vi "rszvl Initiate.vi"(8 "error in (no error)":errorcluster, 9 "Timeout (15000)":u32=15000, 10 "Channel (1)":i32=1, 11 "VISA resource name":refnum<visa-resource-name>) -> (0 "error out":errorcluster, 3 "VISA resource name out":refnum<visa-resource-name>)   [LabVIEW 2014]
doc: "This VI initiates an acquisition. After calling this VI, the spectrum analyzer leaves the idle state and waits for a trigger.\n\nThis VI does not check the instrument status. Typically, the end-user calls this VI only in a sequence of calls to other low-level driver VIs. The sequence performs one operation. The end-user uses the low-level VIs to optimize one or more aspects of interaction with the instrument.\n\nNotes:\n\n(1) Call the Error Query VI at the conclusion of the sequence to check the instrument status.\n\nAttribute(s):\nRSZVL_ATTR_NWA_INIT\n\nRemote-control command(s):\nINITiate<Ch>[:IMMediate]\n*OPC"
uses:
  Instance           3 22Saved   rszvl Initiate .vi
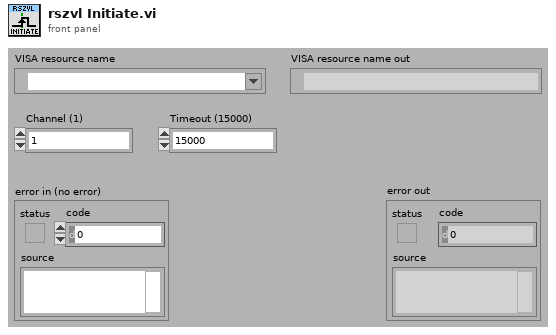
[diagram p1: front panel]
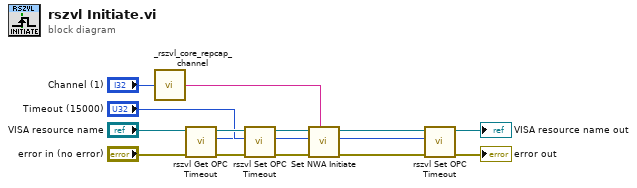
[diagram p0: block diagram]
diagram:
  n1 = call "_rszvl_core_repcap_channel.vi"("Channel"="Channel (1)") -> ("Rep cap"=w2:string)
  n2 = call "rszvl Get OPC Timeout.vi"("error in (no error)"="error in (no error)", "VISA resource name"="VISA resource name") -> ("error out"=w11:errorcluster, "OPC Timeout"=w1:i32, "VISA resource name out"=w12:refnum<visa-resource-name>)  [unwired: 7 in]
  n3 = call "rszvl Set OPC Timeout.vi"("error in (no error)"=w11, "OPC Timeout (15000)"="Timeout (15000)", "VISA resource name"=w12) -> ("error out"=w9:errorcluster, "VISA resource name out"=w10:refnum<visa-resource-name>)  [unwired: 7 in]
  n4 = call "Set NWA Initiate"("Repeated Capabilities"=w2, "error in (no error)"=w9, "instrument handle"=w10) -> ("error out"=w6:errorcluster, "instrument handle out"=w7:refnum<visa-resource-name>)  [unwired: 7 in]
  n5 = call "rszvl Set OPC Timeout.vi"("error in (no error)"=w6, "OPC Timeout (15000)"=w1, "VISA resource name"=w7) -> ("error out"=→"error out":errorcluster, "VISA resource name out"=→"VISA resource name out":refnum<visa-resource-name>)  [unwired: 7 in]
